vi "Drive_Vi.vi"(8 "Yaw":dbl format="%#_13g", 9 "Z":dbl format="%#_13g", 10 "Y":dbl format="%#_13g", 11 "X":dbl format="%#_13g") -> ()   [LabVIEW 2020]
uses:
  <vilib>/addons/control/pid/NI_PID_pid.lvlib
  <vilib>/addons/control/pid/pid.llb/PID (DBL).vi
  <vilib>/Rock Robotics/WPI/ThirdParty/Phoenix-LabVIEW/Motor Controller/Controls/CTRE_Phoenix_MotorControl_ControlMode.ctl
  <vilib>/Rock Robotics/WPI/ThirdParty/Phoenix-LabVIEW/CANCoder/Get/CTRE_Phoenix_CANcoder_GetSensorData.vi
panel:
  out "frontrightmotor":dbl
  out "frontleftdrive":dbl
  in  "PID gains 4":T1={"proportional gain (Kc)"=-0.005, "integral time (Ti, min)"=0.0, "derivative time (Td, min)"=2e-05} {"derivative time (Td, min)" format="%.6f"; "integral time (Ti, min)" format="%.6f"; "proportional gain (Kc)" format="%.6f"}
  in  "PID gains 3":T1={"proportional gain (Kc)"=0.005, "integral time (Ti, min)"=0.0, "derivative time (Td, min)"=2e-05} {"derivative time (Td, min)" format="%.6f"; "integral time (Ti, min)" format="%.6f"; "proportional gain (Kc)" format="%.6f"}
  in  "PID gains 2":T1={"proportional gain (Kc)"=-0.005, "integral time (Ti, min)"=0.0, "derivative time (Td, min)"=2e-05} {"derivative time (Td, min)" format="%.6f"; "integral time (Ti, min)" format="%.6f"; "proportional gain (Kc)" format="%.6f"}
  in  "PID gains":T1={"proportional gain (Kc)"=0.005, "integral time (Ti, min)"=0.0, "derivative time (Td, min)"=2e-05} {"derivative time (Td, min)" format="%.6f"; "integral time (Ti, min)" format="%.6f"; "proportional gain (Kc)" format="%.6f"}
  out "Motor out 4":dbl
  out "Desired Position 4":dbl
  out "Motor out 1":dbl
  out "Desired Position 1":dbl
  out "Motor Out 2":dbl
  out "Desired Position 2":dbl
  out "Motor out 3":dbl
  out "Desired Position 3":dbl
  out "Sensor Position 4":dbl
  out "Sensor Position 3":dbl
  out "Sensor Position 2":dbl
  out "Sensor Position 1":dbl
  out "Rotation steering angle 4":dbl
  out "WheelDirection4":dbl(knob) scale=180.0..-180.0
  out "Throttle 4":dbl(slide) scale=-1.0..1.0
  out "Y4":dbl
  out "X4":dbl
  out "Rotation steering angle 3":dbl
  out "WheelDirection3":dbl(knob) scale=180.0..-180.0
  out "Throttle 3":dbl(slide) scale=-1.0..1.0
  out "Y3":dbl
  out "X3":dbl
  out "Rotation steering angle 2":dbl
  out "WheelDirection2":dbl(knob) scale=180.0..-180.0
  out "Throttle 2":dbl(slide) scale=-1.0..1.0
  out "Y2":dbl
  out "X2":dbl
  out "Rotation steering angle 1":dbl
  out "WheelDirection1":dbl(knob) scale=180.0..-180.0
  out "Throttle 1":dbl(slide) scale=-1.0..1.0
  out "Y1":dbl
  out "X1":dbl
  out "Z - Axis":dbl
  out "Y - Axis":dbl
  out "X - Axis":dbl
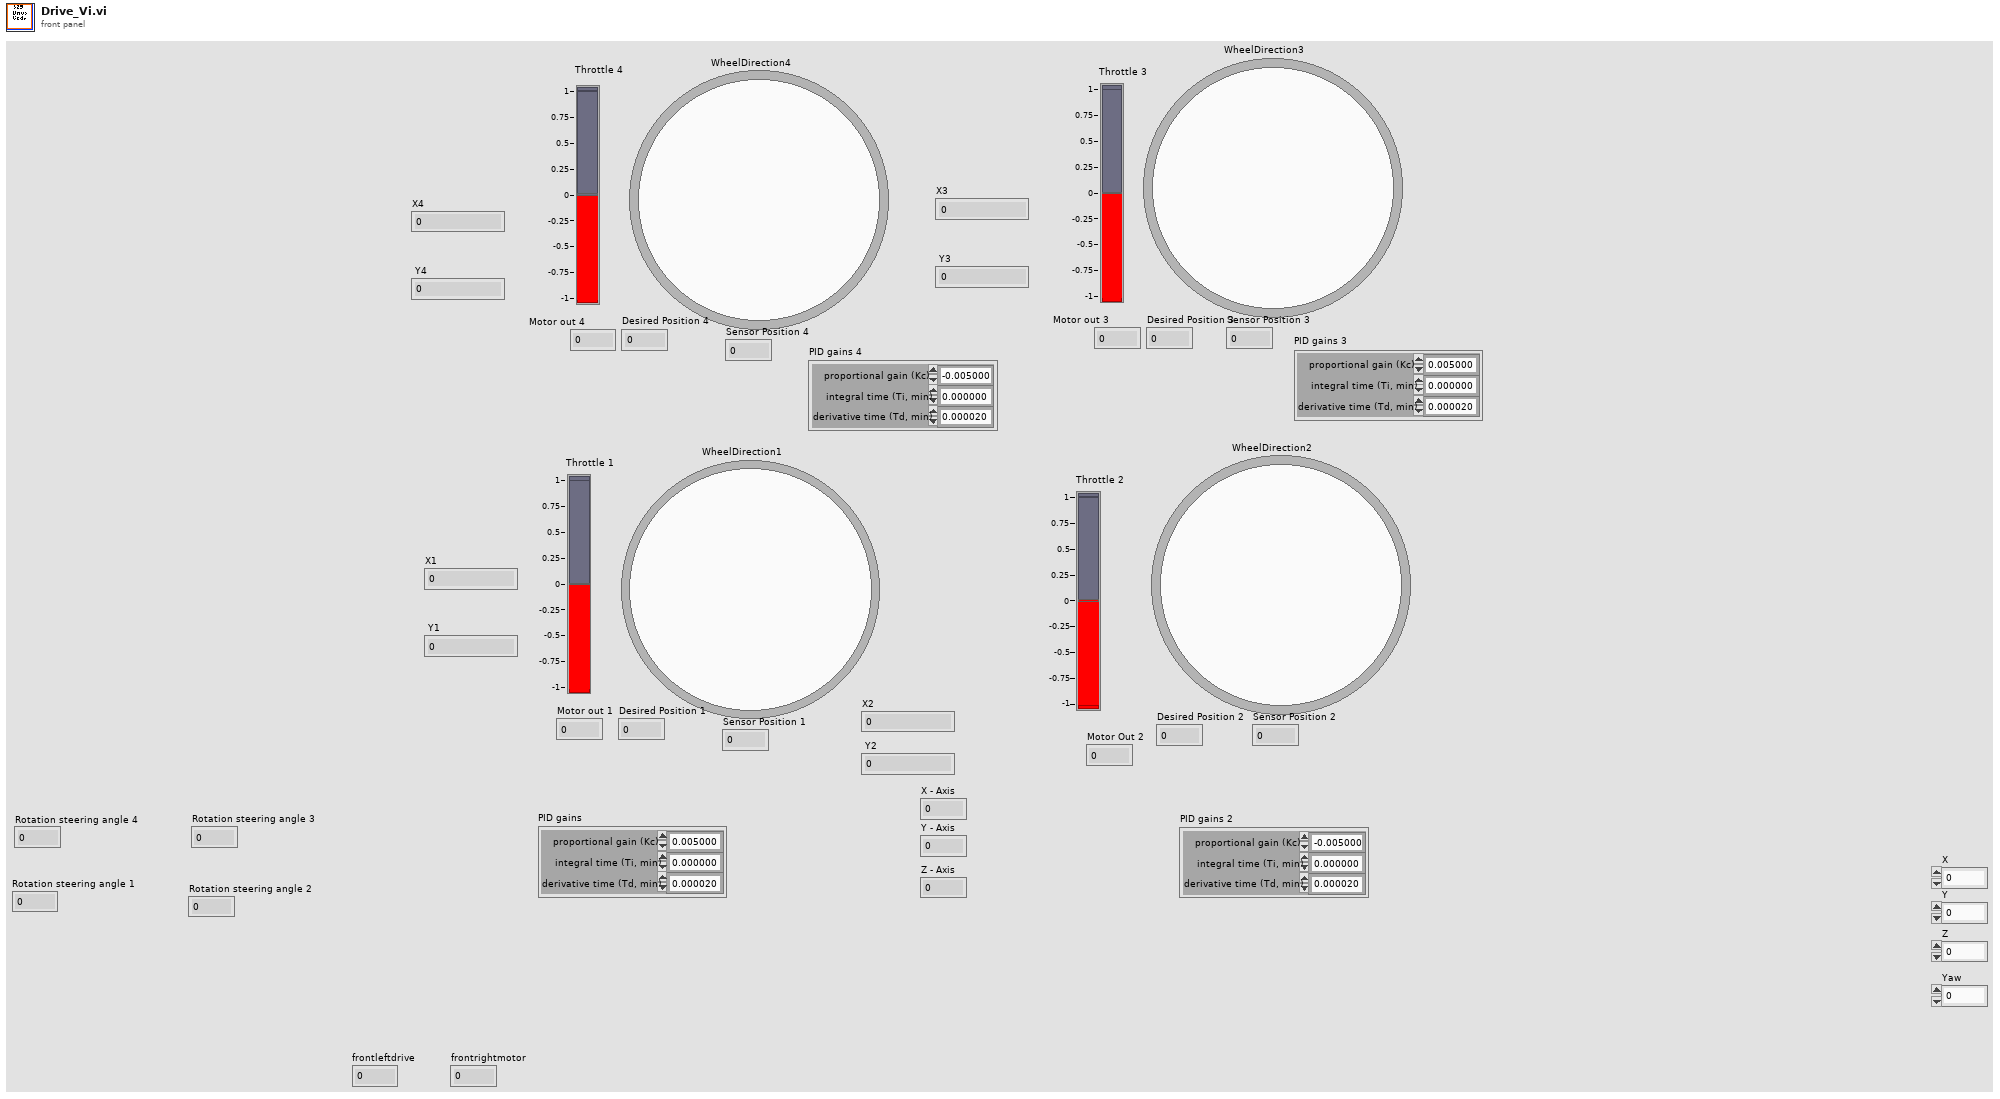
[diagram p1: front panel]
types:
  T1 = cluster{"proportional gain (Kc)":dbl, "integral time (Ti, min)":dbl, "derivative time (Td, min)":dbl}
  T2 = typedef "CTRE_Phoenix_MotorControl_ControlMode.ctl" = u16
  T3 = typedef "WPI_MotorControlDeviceRef.ctl" = cluster{"DeviceStatus":errorcluster, "Type":T4, "PWM":cluster{"PWM Channel":T5, "DeadBand":T6}, "CAN":cluster{"Device Number":u8, "SetOutput VI Ref":variant, "GetOutput VI Ref":variant, "Enable VI Ref":variant, "Disable VI Ref":variant, "Data":variant}, "Invert":bool, "DIO PWM":cluster{"PWM \"Enable\" Channel":T5, "DIOChannel":T7, "PWM Rate":dbl}}
  T4 = typedef "WPI_MotorControlType.ctl" = enum16{"PWM", "CAN", "DIO PWM"}
  T5 = typedef "FPGA_DIOPWMChannel.ctl" = enum8{"PWM 0", "PWM 1", "PWM 2", "PWM 3", "PWM 4", "PWM 5", "PWM 6", "PWM 7", "PWM 8", "PWM 9", "PWM MXP 0", "PWM MXP 1", "PWM MXP 2", "PWM MXP 3", "PWM MXP 4", "PWM MXP 5", "PWM MXP 6", "PWM MXP 7", "PWM MXP 8", "PWM MXP 9", "Invalid"}
  T6 = typedef "WPI_PWMDeadband.ctl" = cluster{"Name":string, "maxPositivePwm":i32, "minPositivePwm":i32, "centerPwm":i32, "maxNegativePwm":i32, "minNegativePwm":i32, "angularRange":u16}
  T7 = typedef "FPGA_DIOChannel.ctl" = enum8{"DIO 0", "DIO 1", "DIO 2", "DIO 3", "DIO 4", "DIO 5", "DIO 6", "DIO 7", "DIO 8", "DIO 9", "DIO MXP 0", "DIO MXP 1", "DIO MXP 2", "DIO MXP 3", "DIO MXP 4", "DIO MXP 5", "DIO MXP 6", "DIO MXP 7", "DIO MXP 8", "DIO MXP 9", "DIO MXP 10", "DIO MXP 11", "DIO MXP 12", "DIO MXP 13", "DIO MXP 14", "DIO MXP 15", "SPI Port CS1", "SPI Port CS2", "SPI Port CS3", "SPI Port MISO", "SPI Port MOSI", "Invalid"}
  T8 = typedef "CTRE_Phoenix_CANcoder_DeviceRef.ctl" = cluster{"DeviceStatus":errorcluster, "Device Number":u8, "Handle":u64, "UsageFrame":u32, "Library Path":path}
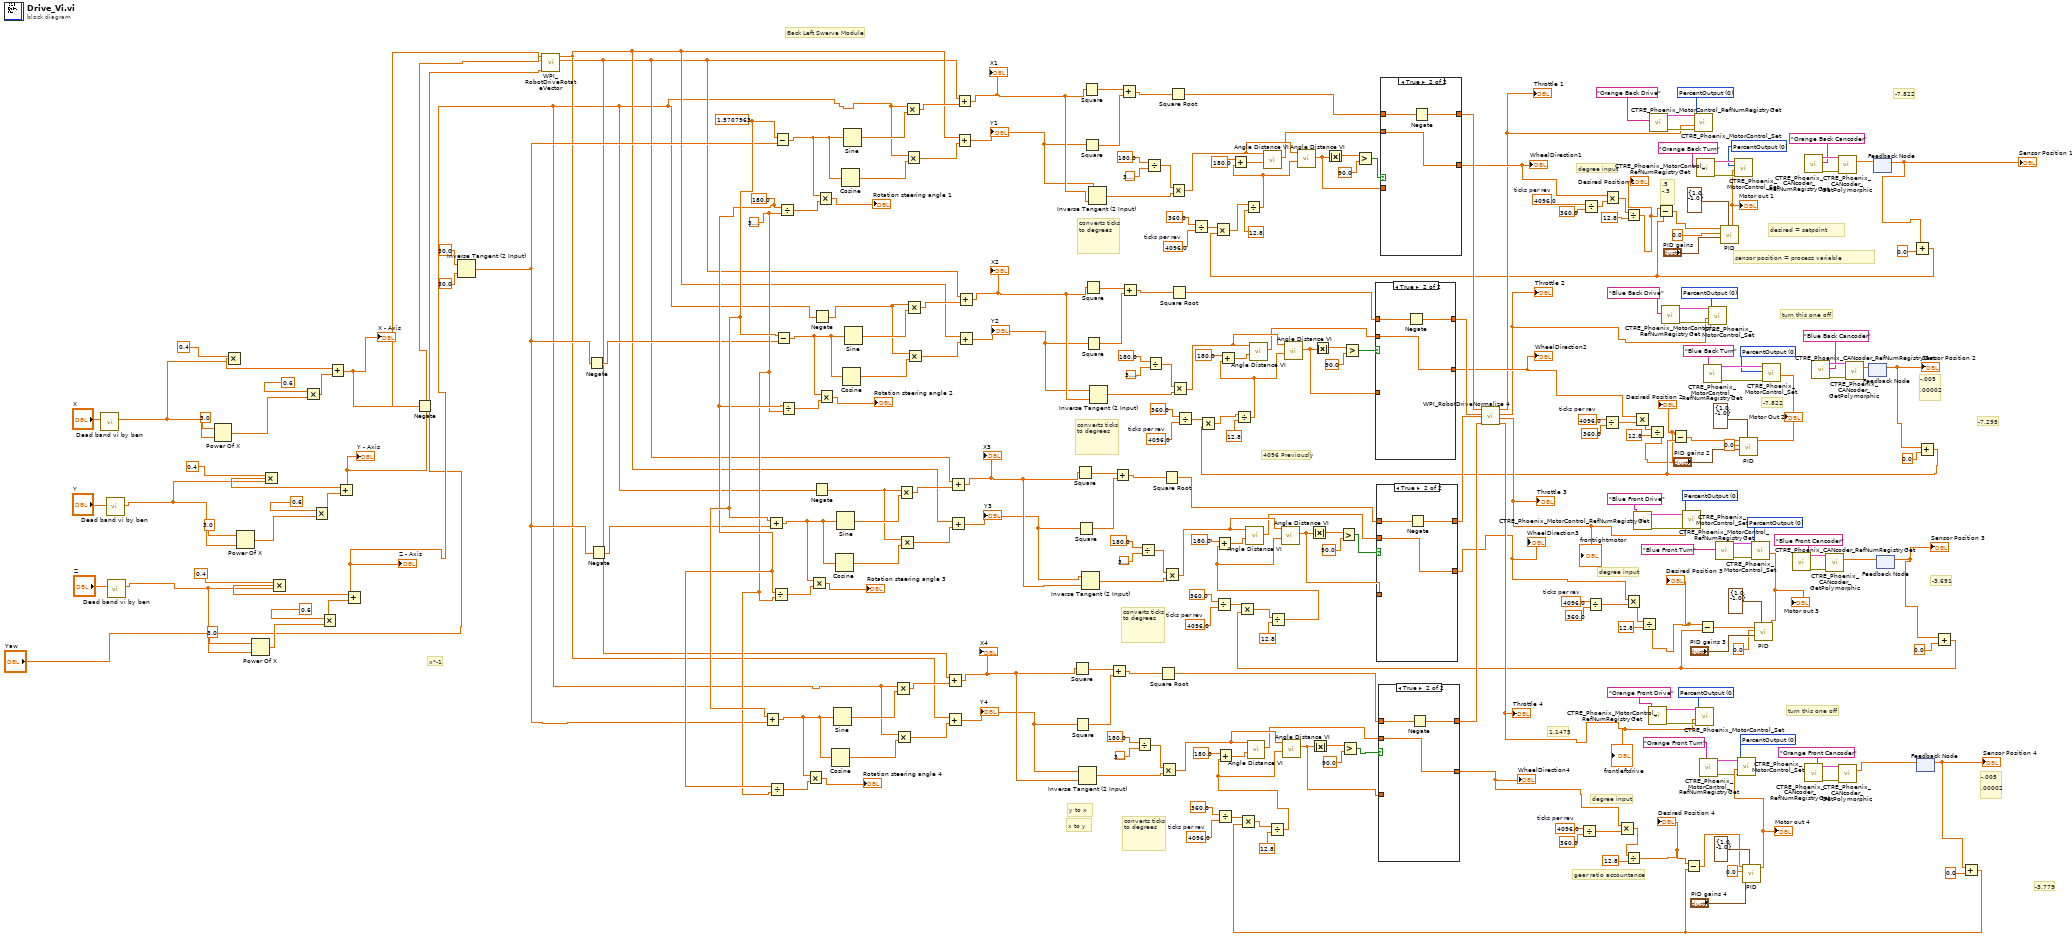
[diagram p0: block diagram]
diagram:
  w101 = T2 0 items=["PercentOutput"=0, "Position"=1, "Velocity"=2, "Current"=3, "Follower"=5, "MotionProfile"=6, "MotionMagic"=7, "MotionProfileArc"=10, "Disabled"=15] ("Control Mode")
  w113 = T2 0 items=["PercentOutput"=0, "Position"=1, "Velocity"=2, "Current"=3, "Follower"=5, "MotionProfile"=6, "MotionMagic"=7, "MotionProfileArc"=10, "Disabled"=15] ("Control Mode")
  w114 = T2 0 items=["PercentOutput"=0, "Position"=1, "Velocity"=2, "Current"=3, "Follower"=5, "MotionProfile"=6, "MotionMagic"=7, "MotionProfileArc"=10, "Disabled"=15] ("Control Mode")
  w115 = T2 0 items=["PercentOutput"=0, "Position"=1, "Velocity"=2, "Current"=3, "Follower"=5, "MotionProfile"=6, "MotionMagic"=7, "MotionProfileArc"=10, "Disabled"=15] ("Control Mode")
  w116 = T2 0 items=["PercentOutput"=0, "Position"=1, "Velocity"=2, "Current"=3, "Follower"=5, "MotionProfile"=6, "MotionMagic"=7, "MotionProfileArc"=10, "Disabled"=15] ("Control Mode")
  w117 = T2 0 items=["PercentOutput"=0, "Position"=1, "Velocity"=2, "Current"=3, "Follower"=5, "MotionProfile"=6, "MotionMagic"=7, "MotionProfileArc"=10, "Disabled"=15] ("Control Mode")
  w118 = T2 0 items=["PercentOutput"=0, "Position"=1, "Velocity"=2, "Current"=3, "Follower"=5, "MotionProfile"=6, "MotionMagic"=7, "MotionProfileArc"=10, "Disabled"=15] ("Control Mode")
  w119 = T2 0 items=["PercentOutput"=0, "Position"=1, "Velocity"=2, "Current"=3, "Follower"=5, "MotionProfile"=6, "MotionMagic"=7, "MotionProfileArc"=10, "Disabled"=15] ("Control Mode")
  w131 = 4096.0  # ticks per rev
  w143 = 4096.0  # ticks per rev
  w157 = 4096.0  # ticks per rev
  w168 = 4096.0  # ticks per rev
  w64 = 1.5707963 ("y")
  w177 = 4096.0  # ticks per rev
  w181 = 4096.0  # ticks per rev
  w185 = 4096.0  # ticks per rev
  w104 = 4096.0  # ticks per rev
  w62 = 3.141592653589793
  w63 = 180.0 ("x")
  # "4096 Previously"
  # "x*-1"
  # ".5\n-.5"
  # "y to x"
  # "x to y"
  # "sensor position = process variable"
  # "desired = setpoint"
  # "-.005\n\n.00002"
  # "-.005\n\n.00002"
  # "-7.822"
  # "-7.295"
  # "-3.691"
  # "-3.779"
  # "1.1475"
  # "turn this one off"
  # "turn this one off"
  # "gear ratio accountance"
  # "converts ticks to degrees"
  # "converts ticks to degrees"
  # "converts ticks to degrees"
  # "converts ticks to degrees"
  # "degree input"
  # "degree input"
  # "degree input"
  # "Back Left Swerve Module"
  # "-7.822"
  n1 = call "Dead band vi by ben.vi"("Numeric"="X") -> ("Deadbanded Value"=w275:dbl)  [unwired: 10 in]
  n2 = call "Dead band vi by ben.vi"("Numeric"="Y") -> ("Deadbanded Value"=w268:dbl)  [unwired: 10 in]
  n3 = call "Dead band vi by ben.vi"("Numeric"="Z") -> ("Deadbanded Value"=w261:dbl)  [unwired: 10 in]
  n4 = Power Of X(1:w275, 2:3.0 ("y")) -> (0:w279:dbl)
  n5 = Multiply(x=0.4, y=w275) -> (x*y=w276:dbl)
  n6 = Power Of X(1:w268, 2:3.0 ("y")) -> (0:w272:dbl)
  n7 = Power Of X(1:w261, 2:3.0 ("y")) -> (0:w265:dbl)
  n8 = Multiply(x=0.4, y=w268) -> (x*y=w269:dbl)
  n9 = Multiply(x=0.4, y=w261) -> (x*y=w262:dbl)
  n10 = Multiply(x=0.6, y=w279) -> (x*y=w277:dbl)
  n11 = Multiply(x=0.6, y=w272) -> (x*y=w270:dbl)
  n12 = Multiply(x=0.6, y=w265) -> (x*y=w263:dbl)
  n13 = Add(x=w276, y=w277) -> (x+y=w7:dbl)
  "X - Axis" <- w7
  n14 = Add(x=w269, y=w270) -> (x+y=w6:dbl)
  "Y - Axis" <- w6
  n15 = Add(x=w262, y=w263) -> (x+y=w9:dbl)
  "Z - Axis" <- w9
  n16 = Negate(x=w7) -> (-x=w5:dbl)
  n17 = Inverse Tangent (2 Input)(1:30.0 ("x"), 2:30.0 ("y")) -> (0:w54:dbl)
  n18 = call <vilib>:"WPI_RobotDriveRotateVector.vi"("Angle"="Yaw", "X"=w5, "Y"=w6) -> ("X'"=w12:dbl, "Y'"=w13:dbl)  [unwired: 7 out]
  n19 = Negate(x=w54) -> (-x=w55:dbl)
  n20 = Negate(x=w54) -> (-x=w53:dbl)
  n21 = Add(x=w64, y=w54) -> (x+y=w212:dbl)
  n22 = Add(x=w64, y=w53) -> (x+y=w225:dbl)
  n23 = Divide(x=w63, y=w62) -> (x/y=w211:dbl)
  n24 = Divide(x=w63, y=w62) -> (x/y=w224:dbl)
  n25 = Subtract(x=w64, y=w54) -> (x-y=w253:dbl)
  n26 = Subtract(x=w64, y=w55) -> (x-y=w239:dbl)
  n27 = Divide(x=w63, y=w62) -> (x/y=w252:dbl)
  n28 = Divide(x=w63, y=w62) -> (x/y=w238:dbl)
  n29 = Multiply(x=w212, y=w211) -> (x*y=→"Rotation steering angle 4":dbl)
  n30 = Multiply(x=w225, y=w224) -> (x*y=→"Rotation steering angle 3":dbl)
  n31 = Negate(x=w9) -> (-x=w10:dbl)
  n32 = Negate(x=w9) -> (-x=w11:dbl)
  n33 = Multiply(x=w253, y=w252) -> (x*y=→"Rotation steering angle 1":dbl)
  n34 = Multiply(x=w239, y=w238) -> (x*y=→"Rotation steering angle 2":dbl)
  n35 = Cosine(x=w212) -> (cos(x)=w210:dbl)
  n36 = Sine(x=w212) -> (sin(x)=w209:dbl)
  n37 = Cosine(x=w225) -> (cos(x)=w223:dbl)
  n38 = Sine(x=w225) -> (sin(x)=w222:dbl)
  n39 = Cosine(x=w253) -> (cos(x)=w250:dbl)
  n40 = Cosine(x=w239) -> (cos(x)=w236:dbl)
  n41 = Sine(x=w253) -> (sin(x)=w249:dbl)
  n42 = Sine(x=w239) -> (sin(x)=w235:dbl)
  n43 = Multiply(x=w9, y=w209) -> (x*y=w208:dbl)
  n44 = Multiply(x=w9, y=w210) -> (x*y=w207:dbl)
  n45 = Multiply(x=w10, y=w222) -> (x*y=w221:dbl)
  n46 = Multiply(x=w10, y=w223) -> (x*y=w220:dbl)
  n47 = Multiply(x=w9, y=w249) -> (x*y=w248:dbl)
  n48 = Multiply(x=w9, y=w250) -> (x*y=w247:dbl)
  n49 = Multiply(x=w11, y=w235) -> (x*y=w234:dbl)
  n50 = Multiply(x=w11, y=w236) -> (x*y=w233:dbl)
  n51 = Add(x=w12, y=w208) -> (x+y=w16:dbl)
  "X4" <- w16
  n52 = Add(x=w13, y=w207) -> (x+y=w15:dbl)
  "Y4" <- w15
  n53 = Add(x=w12, y=w221) -> (x+y=w18:dbl)
  "X3" <- w18
  n54 = Add(x=w13, y=w220) -> (x+y=w17:dbl)
  "Y3" <- w17
  n55 = Add(x=w12, y=w248) -> (x+y=w23:dbl)
  "X1" <- w23
  n56 = Add(x=w13, y=w247) -> (x+y=w22:dbl)
  "Y1" <- w22
  n57 = Add(x=w12, y=w234) -> (x+y=w25:dbl)
  "X2" <- w25
  n58 = Add(x=w13, y=w233) -> (x+y=w24:dbl)
  "Y2" <- w24
  n59 = Square(x=w16) -> (x^2=w219:dbl)
  n60 = Square(x=w15) -> (x^2=w217:dbl)
  n61 = Square(x=w18) -> (x^2=w232:dbl)
  n62 = Square(x=w17) -> (x^2=w230:dbl)
  n63 = Inverse Tangent (2 Input)(1:w16, 2:w15) -> (0:w215:dbl)
  n64 = Inverse Tangent (2 Input)(1:w18, 2:w17) -> (0:w228:dbl)
  n65 = Square(x=w23) -> (x^2=w260:dbl)
  n66 = Square(x=w22) -> (x^2=w258:dbl)
  n67 = Square(x=w25) -> (x^2=w246:dbl)
  n68 = Square(x=w24) -> (x^2=w244:dbl)
  n69 = Inverse Tangent (2 Input)(1:w23, 2:w22) -> (0:w256:dbl)
  n70 = Inverse Tangent (2 Input)(1:w25, 2:w24) -> (0:w242:dbl)
  n71 = Add(x=w219, y=w217) -> (x+y=w218:dbl)
  n72 = Add(x=w232, y=w230) -> (x+y=w231:dbl)
  n73 = Add(x=w260, y=w258) -> (x+y=w259:dbl)
  n74 = Add(x=w246, y=w244) -> (x+y=w245:dbl)
  n75 = Divide(x=180.0, y=3.141592653589793) -> (x/y=w216:dbl)
  n76 = Divide(x=180.0, y=3.141592653589793) -> (x/y=w229:dbl)
  n77 = Divide(x=180.0, y=3.141592653589793) -> (x/y=w257:dbl)
  n78 = Divide(x=180.0, y=3.141592653589793) -> (x/y=w243:dbl)
  n79 = Square Root(x=w218) -> (sqrt(x)=w126:dbl)
  n80 = Multiply(x=w216, y=w215) -> (x*y=w127:dbl)
  n81 = Square Root(x=w231) -> (sqrt(x)=w137:dbl)
  n82 = Multiply(x=w229, y=w228) -> (x*y=w139:dbl)
  n83 = Square Root(x=w259) -> (sqrt(x)=w162:dbl)
  n84 = Multiply(x=w257, y=w256) -> (x*y=w167:dbl)
  n85 = Square Root(x=w245) -> (sqrt(x)=w150:dbl)
  n86 = Multiply(x=w243, y=w242) -> (x*y=w153:dbl)
  n87 = Divide(x=360.0 ("y"), y=w157) -> (x/y=w156:dbl)
  n88 = Divide(x=360.0 ("y"), y=w168) -> (x/y=w103:dbl)
  n89 = Divide(x=360.0 ("y"), y=w143) -> (x/y=w142:dbl)
  n90 = Divide(x=360.0 ("y"), y=w131) -> (x/y=w130:dbl)
  n91 = Divide(x=w177, y=360.0) -> (x/y=w178:dbl)
  n92 = Divide(x=w104, y=360.0) -> (x/y=w189:dbl)
  n93 = Divide(x=w181, y=360.0) -> (x/y=w182:dbl)
  n94 = Divide(x=w185, y=360.0) -> (x/y=w186:dbl)
  n95 = call <vilib>:"CTRE_Phoenix_MotorControl_RefNumRegistryGet.vi"("refnum name"="Blue Front Drive") -> ("error out"=w110:errorcluster, "PhoenixMotorControlDevRef"=w202:T3)  [unwired: 9 in]
  n96 = call <vilib>:"CTRE_Phoenix_MotorControl_RefNumRegistryGet.vi"("refnum name"="Orange Front Drive") -> ("error out"=w109:errorcluster, "PhoenixMotorControlDevRef"=w199:T3)  [unwired: 9 in]
  n97 = call <vilib>:"CTRE_Phoenix_MotorControl_RefNumRegistryGet.vi"("refnum name"="Orange Back Drive") -> ("error out"=w112:errorcluster, "PhoenixMotorControlDevRef"=w206:T3)  [unwired: 9 in]
  n98 = call <vilib>:"CTRE_Phoenix_MotorControl_RefNumRegistryGet.vi"("refnum name"="Blue Back Drive") -> ("error out"=w111:errorcluster, "PhoenixMotorControlDevRef"=w203:T3)  [unwired: 9 in]
  n99 = call <vilib>:"CTRE_Phoenix_MotorControl_RefNumRegistryGet.vi"("refnum name"="Orange Back Turn") -> ("error out"=w108:errorcluster, "PhoenixMotorControlDevRef"=w197:T3)  [unwired: 9 in]
  n100 = call <vilib>:"CTRE_Phoenix_MotorControl_RefNumRegistryGet.vi"("refnum name"="Orange Front Turn") -> ("error out"=w105:errorcluster, "PhoenixMotorControlDevRef"=w194:T3)  [unwired: 9 in]
  n101 = call <vilib>:"CTRE_Phoenix_MotorControl_RefNumRegistryGet.vi"("refnum name"="Blue Back Turn") -> ("error out"=w107:errorcluster, "PhoenixMotorControlDevRef"=w196:T3)  [unwired: 9 in]
  n102 = call <vilib>:"CTRE_Phoenix_MotorControl_RefNumRegistryGet.vi"("refnum name"="Blue Front Turn") -> ("error out"=w106:errorcluster, "PhoenixMotorControlDevRef"=w195:T3)  [unwired: 9 in]
  n103 = call <vilib>:"CTRE_Phoenix_CANcoder_RefNumRegistryGet.vi"("refnum name"="Blue Front Cancoder") -> ("error out"=w93:errorcluster, "CTRE_CANcoder_DeviceRef"=w94:T8)  [unwired: 9 in]
  n104 = call <vilib>:"CTRE_Phoenix_CANcoder_RefNumRegistryGet.vi"("refnum name"="Orange Back Cancoder") -> ("error out"=w99:errorcluster, "CTRE_CANcoder_DeviceRef"=w100:T8)  [unwired: 9 in]
  n105 = call <vilib>:"CTRE_Phoenix_CANcoder_RefNumRegistryGet.vi"("refnum name"="Orange Front Cancoder") -> ("error out"=w90:errorcluster, "CTRE_CANcoder_DeviceRef"=w91:T8)  [unwired: 9 in]
  n106 = call <vilib>:"CTRE_Phoenix_CANcoder_RefNumRegistryGet.vi"("refnum name"="Blue Back Cancoder") -> ("error out"=w96:errorcluster, "CTRE_CANcoder_DeviceRef"=w97:T8)  [unwired: 9 in]
  n107 = call-poly <vilib>:"CTRE_Phoenix_CANcoder_GetPolymorphic.vi"("CTRE_CANcoder_DeviceRef"=w94, "error in"=w93) -> ("Position"=w66:dbl)  [unwired: 9 in, 4 out]
  n108 = call-poly <vilib>:"CTRE_Phoenix_CANcoder_GetPolymorphic.vi"("CTRE_CANcoder_DeviceRef"=w100, "error in"=w99) -> ("Position"=w51:dbl)  [unwired: 9 in, 4 out]
  n109 = call-poly <vilib>:"CTRE_Phoenix_CANcoder_GetPolymorphic.vi"("CTRE_CANcoder_DeviceRef"=w91, "error in"=w90) -> ("Position"=w65:dbl)  [unwired: 9 in, 4 out]
  n110 = call-poly <vilib>:"CTRE_Phoenix_CANcoder_GetPolymorphic.vi"("CTRE_CANcoder_DeviceRef"=w97, "error in"=w96) -> ("Position"=w67:dbl)  [unwired: 9 in, 4 out]
  n111 = feedback #1() -> (w50:dbl)  [unwired: 1 in]
  "Sensor Position 2" <- w50
  n112 = feedback-in #1(w67) -> ()
  n113 = feedback #2() -> (w40:dbl)  [unwired: 1 in]
  "Sensor Position 1" <- w40
  n114 = feedback-in #2(w51) -> ()
  n115 = feedback #3() -> (w48:dbl)  [unwired: 1 in]
  "Sensor Position 3" <- w48
  n116 = feedback-in #3(w66) -> ()
  n117 = Add(x=w40, y=0.0) -> (x+y=w36:dbl)
  n118 = Multiply(x=w103, y=w36) -> (x*y=w57:dbl)
  n119 = Divide(x=w57, y=12.8 ("x")) -> (x/y=w83:dbl)
  n120 = Add(x=180.0, y=w83) -> (x+y=w171:dbl)
  n121 = call "Angle Distance VI.vi"("current angle"=w171, "target angle"=w167) -> ("distance"=w163:dbl)  [unwired: 9 in]
  n122 = call "Angle Distance VI.vi"("current angle"=w83, "target angle"=w167) -> ("distance"=w164:dbl)  [unwired: 9 in]
  n123 = Absolute Value(x=w164) -> (abs(x)=w166:dbl)
  n124 = Greater?(x=w166, y=90.0 ("x")) -> (0:w88:bool)
  n125 = case shown="True" w88 {
    tunnel: w164 -> [w283 _]
    tunnel: [w283 w286] -> w102
    tunnel: w163 -> [_ w286]
    tunnel: w162 -> [w282 w285]
    tunnel: [w282 w284] -> w161
    frame False {
    }
    frame True {
      n126 = Negate(x=w285) -> (-x=w284:dbl)
    }
  }
  "WheelDirection1" <- w102
  n127 = Multiply(x=w102, y=w189) -> (x*y=w85:dbl)
  n128 = Divide(x=w85, y=12.8) -> (x/y=w21:dbl)
  "Desired Position 1" <- w21
  n129 = Subtract(x=w21, y=w36) -> (x-y=w35:dbl)
  n130 = call-poly <vilib>:"PID.vi"("output range"=cluster{"output high":dbl, "output low":dbl} {"output high"=1.0, "output low"=-1.0}, "PID gains"="PID gains", "process variable"=0.0, "setpoint"=w35) -> ("output"=w39:dbl)  [unwired: 6 in, 1 out]
  "Motor out 1" <- w39
  n131 = call <vilib>:"CTRE_Phoenix_MotorControl_Set.vi"("error in (no error)"=w108, "Output"=w39, "Control Mode"=w101, "PhoenixMotorControlDevRef"=w197) -> ()  [unwired: 6 in, 2 out]
  n132 = feedback #4() -> (w45:dbl)  [unwired: 1 in]
  "Sensor Position 4" <- w45
  n133 = feedback-in #4(w65) -> ()
  n134 = Add(x=w50, y=0.0) -> (x+y=w34:dbl)
  n135 = Multiply(x=w156, y=w34) -> (x*y=w75:dbl)
  n136 = Divide(x=w75, y=12.8) -> (x/y=w74:dbl)
  n137 = Add(x=180.0, y=w74) -> (x+y=w160:dbl)
  n138 = call "Angle Distance VI.vi"("current angle"=w160, "target angle"=w153) -> ("distance"=w151:dbl)  [unwired: 9 in]
  n139 = call "Angle Distance VI.vi"("current angle"=w74, "target angle"=w153) -> ("distance"=w148:dbl)  [unwired: 9 in]
  n140 = Absolute Value(x=w148) -> (abs(x)=w155:dbl)
  n141 = Greater?(x=w155, y=90.0 ("x")) -> (0:w152:bool)
  n142 = case shown="True" w152 {
    tunnel: w148 -> [w288 _]
    tunnel: [w288 w291] -> w147
    tunnel: w151 -> [_ w291]
    tunnel: w150 -> [w287 w290]
    tunnel: [w287 w289] -> w149
    frame False {
    }
    frame True {
      n143 = Negate(x=w290) -> (-x=w289:dbl)
    }
  }
  "WheelDirection2" <- w147
  n144 = Multiply(x=w147, y=w186) -> (x*y=w81:dbl)
  n145 = Divide(x=w81, y=12.8) -> (x/y=w20:dbl)
  "Desired Position 2" <- w20
  n146 = Subtract(x=w20, y=w34) -> (x-y=w33:dbl)
  n147 = call-poly <vilib>:"PID.vi"("output range"=cluster{"output high":dbl, "output low":dbl} {"output high"=1.0, "output low"=-1.0}, "PID gains"="PID gains 2", "process variable"=0.0, "setpoint"=w33) -> ("output"=w173:dbl)  [unwired: 6 in, 1 out]
  "Motor Out 2" <- w173
  n148 = call <vilib>:"CTRE_Phoenix_MotorControl_Set.vi"("error in (no error)"=w107, "Output"=w173, "Control Mode"=w115, "PhoenixMotorControlDevRef"=w196) -> ()  [unwired: 6 in, 2 out]
  n149 = Add(x=w48, y=0.0) -> (x+y=w31:dbl)
  n150 = Multiply(x=w142, y=w31) -> (x*y=w72:dbl)
  n151 = Divide(x=w72, y=12.8) -> (x/y=w71:dbl)
  n152 = Add(x=180.0, y=w71) -> (x+y=w146:dbl)
  n153 = call "Angle Distance VI.vi"("current angle"=w146, "target angle"=w139) -> ("distance"=w138:dbl)  [unwired: 9 in]
  n154 = call "Angle Distance VI.vi"("current angle"=w71, "target angle"=w139) -> ("distance"=w135:dbl)  [unwired: 9 in]
  n155 = Absolute Value(x=w135) -> (abs(x)=w141:dbl)
  n156 = Greater?(x=w141, y=90.0 ("x")) -> (0:w120:bool)
  n157 = case shown="True" w120 {
    tunnel: w135 -> [w293 _]
    tunnel: [w293 w296] -> w14
    tunnel: w138 -> [_ w296]
    tunnel: w137 -> [w292 w295]
    tunnel: [w292 w294] -> w136
    frame False {
    }
    frame True {
      n158 = Negate(x=w295) -> (-x=w294:dbl)
    }
  }
  "WheelDirection3" <- w14
  n159 = Multiply(x=w14, y=w182) -> (x*y=w79:dbl)
  n160 = Divide(x=w79, y=12.8) -> (x/y=w19:dbl)
  "Desired Position 3" <- w19
  n161 = Subtract(x=w19, y=w31) -> (x-y=w30:dbl)
  n162 = call-poly <vilib>:"PID.vi"("output range"=cluster{"output high":dbl, "output low":dbl} {"output high"=1.0, "output low"=-1.0}, "PID gains"="PID gains 3", "process variable"=0.0, "setpoint"=w30) -> ("output"=w174:dbl)  [unwired: 6 in, 1 out]
  "Motor out 3" <- w174
  n163 = call <vilib>:"CTRE_Phoenix_MotorControl_Set.vi"("error in (no error)"=w106, "Output"=w174, "Control Mode"=w116, "PhoenixMotorControlDevRef"=w195) -> ()  [unwired: 6 in, 2 out]
  n164 = Add(x=w45, y=0.0) -> (x+y=w27:dbl)
  n165 = Multiply(x=w130, y=w27) -> (x*y=w69:dbl)
  n166 = Divide(x=w69, y=12.8) -> (x/y=w68:dbl)
  n167 = Add(x=180.0, y=w68) -> (x+y=w134:dbl)
  n168 = call "Angle Distance VI.vi"("current angle"=w134, "target angle"=w127) -> ("distance"=w123:dbl)  [unwired: 9 in]
  n169 = call "Angle Distance VI.vi"("current angle"=w68, "target angle"=w127) -> ("distance"=w122:dbl)  [unwired: 9 in]
  n170 = Absolute Value(x=w122) -> (abs(x)=w129:dbl)
  n171 = Greater?(x=w129, y=90.0 ("x")) -> (0:w124:bool)
  n172 = case shown="True" w124 {
    tunnel: w122 -> [w298 _]
    tunnel: [w298 w301] -> w121
    tunnel: w123 -> [_ w301]
    tunnel: w126 -> [w297 w300]
    tunnel: [w297 w299] -> w125
    frame False {
    }
    frame True {
      n173 = Negate(x=w300) -> (-x=w299:dbl)
    }
  }
  "WheelDirection4" <- w121
  n174 = call <vilib>:"WPI_RobotDriveNormalize 4.vi"("D"=w125, "C"=w136, "B"=w149, "A"=w161) -> ("D'"=w41:dbl, "C'"=w198:dbl, "B'"=w42:dbl, "A'"=w38:dbl)
  "Throttle 1" <- w38
  "Throttle 2" <- w42
  "Throttle 3" <- w198
  "Throttle 4" <- w41
  "frontleftdrive" <- w41
  "frontrightmotor" <- w198
  n175 = Multiply(x=w121, y=w178) -> (x*y=w77:dbl)
  n176 = Divide(x=w77, y=12.8) -> (x/y=w8:dbl)
  "Desired Position 4" <- w8
  n177 = call <vilib>:"CTRE_Phoenix_MotorControl_Set.vi"("error in (no error)"=w110, "Output"=w198, "Control Mode"=w119, "PhoenixMotorControlDevRef"=w202) -> ()  [unwired: 6 in, 2 out]
  n178 = Subtract(x=w8, y=w27) -> (x-y=w26:dbl)
  n179 = call <vilib>:"CTRE_Phoenix_MotorControl_Set.vi"("error in (no error)"=w112, "Output"=w38, "Control Mode"=w113, "PhoenixMotorControlDevRef"=w206) -> ()  [unwired: 6 in, 2 out]
  n180 = call <vilib>:"CTRE_Phoenix_MotorControl_Set.vi"("error in (no error)"=w109, "Output"=w41, "Control Mode"=w118, "PhoenixMotorControlDevRef"=w199) -> ()  [unwired: 6 in, 2 out]
  n181 = call <vilib>:"CTRE_Phoenix_MotorControl_Set.vi"("error in (no error)"=w111, "Output"=w42, "Control Mode"=w114, "PhoenixMotorControlDevRef"=w203) -> ()  [unwired: 6 in, 2 out]
  n182 = call-poly <vilib>:"PID.vi"("output range"=cluster{"output high":dbl, "output low":dbl} {"output high"=1.0, "output low"=-1.0}, "PID gains"="PID gains 4", "process variable"=0.0, "setpoint"=w26) -> ("output"=w172:dbl)  [unwired: 6 in, 1 out]
  "Motor out 4" <- w172
  n183 = call <vilib>:"CTRE_Phoenix_MotorControl_Set.vi"("error in (no error)"=w105, "Output"=w172, "Control Mode"=w117, "PhoenixMotorControlDevRef"=w194) -> ()  [unwired: 6 in, 2 out]
